vi "Error Query.vi"(8 "error in (no error)":errorcluster, 11 "VISA resource name":refnum<visa-resource-name>) -> (0 "error out":errorcluster, 1 "Error Message":string, 2 "Error Code":i32[](array[numeric]), 3 "VISA resource name out":refnum<visa-resource-name>)   [LabVIEW 2018, in "LeCroy Wave Series.lvlib"]
doc: "This VI queries the instrument for any errors in the instrument's error queue. It will continue to read errors until all errors have been read from the instrument. Any errors will be returned in the Error Out cluster.\n\nNote:\nThis VI is called automatically by most driver VIs so it is not usually necessary to call this in an application."
uses:
  LeCroy Wave Series.lvlib
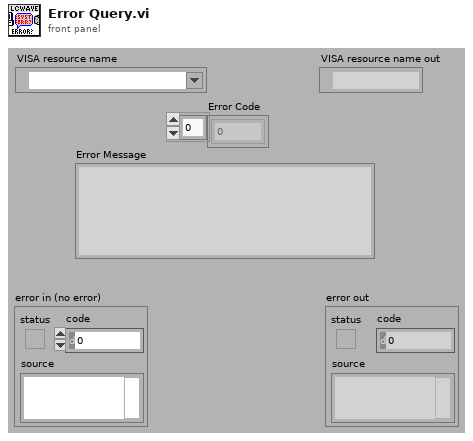
[diagram p1: front panel]
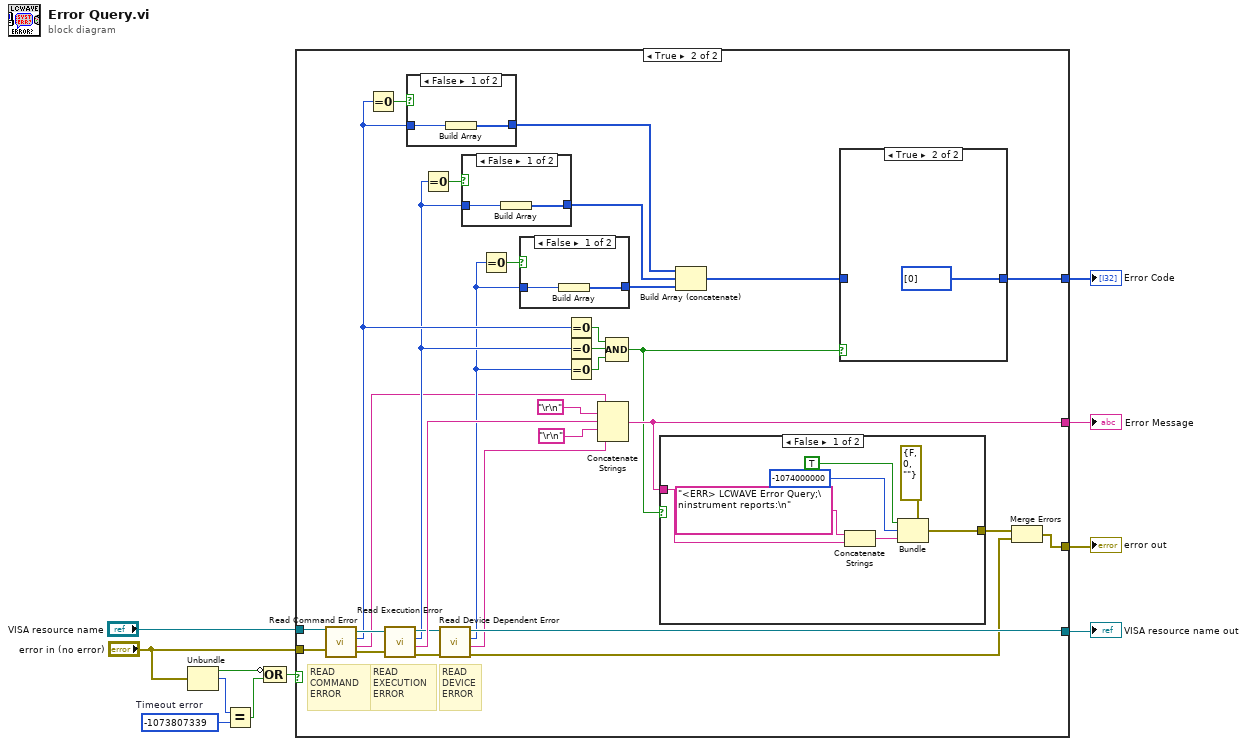
[diagram p0: block diagram]
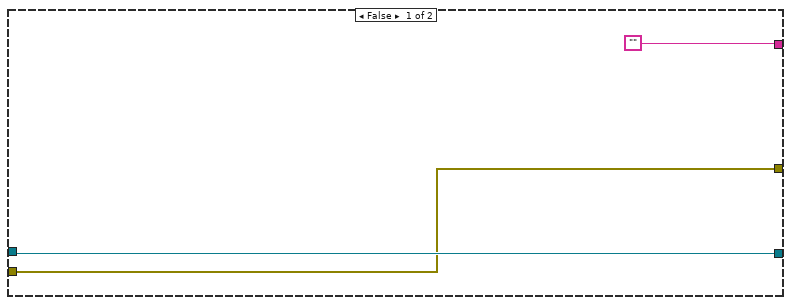
[diagram p2: hidden frame]
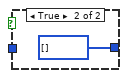
[diagram p4: hidden frame]
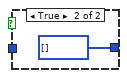
[diagram p5: hidden frame]
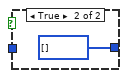
[diagram p6: hidden frame]
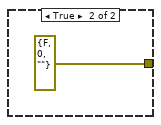
[diagram p7: hidden frame]
diagram:
  w4 = -1073807339  # Timeout error
  n1 = Unbundle("error in (no error)") -> ("status"=w6:bool, "code"=w5:i32)  [unwired: 1 out]
  n2 = Equal?(x=w5, y=w4) -> (x = y?=w3:bool)
  n3 = Compound Arithmetic op=OR(invert w6, w3) -> (w2:bool)
  n4 = case shown="True" w2 {
    tunnel: "VISA resource name" -> [w14 w39]
    tunnel: [w14 w32] -> w10
    tunnel: [w13 w40] -> w9
    tunnel: ["" ("Empty String Constant") w28] -> w8
    tunnel: "error in (no error)" -> [w13 w38]
    tunnel: [_ w17] -> w1
    frame False {
    }
    frame True {
      # "READ\nDEVICE\nERROR"
      # "READ\nEXECUTION\nERROR"
      # "READ\nCOMMAND\nERROR"
      n5 = call "Read Command Error.vi"("error in (no error)"=w38, "VISA resource name"=w39) -> ("error out"=w36:errorcluster, "Error Message"=w15:string, "Error Code"=w26:i32, "VISA resource name out"=w37:refnum<visa-resource-name>)  [unwired: 6 in]
      n6 = Equal To 0?(x=w26) -> (x = 0?=w27:bool)
      n7 = call "Read Execution Error.vi"("error in (no error)"=w36, "VISA resource name"=w37) -> ("error out"=w33:errorcluster, "Error Message"=w35:string, "Error Code"=w24:i32, "VISA resource name out"=w34:refnum<visa-resource-name>)  [unwired: 6 in]
      n8 = case shown="False" w27 {
        tunnel: [w54 i32[] []] -> w20
        tunnel: w26 -> [w55 _]
        frame False {
          n9 = Build Array(w55) -> (w54:i32[])
        }
        frame True {
        }
      }
      n10 = Equal To 0?(x=w24) -> (x = 0?=w25:bool)
      n11 = call "Read Device Dependent Error.vi"("error in (no error)"=w33, "VISA resource name"=w34) -> ("error out"=w31:errorcluster, "Error Message"=w29:string, "Error Code"=w22:i32, "VISA resource name out"=w32:refnum<visa-resource-name>)  [unwired: 6 in]
      n12 = case shown="False" w25 {
        tunnel: [w51 i32[] []] -> w19
        tunnel: w24 -> [w52 _]
        frame False {
          n13 = Build Array(w52) -> (w51:i32[])
        }
        frame True {
        }
      }
      n14 = Equal To 0?(x=w22) -> (x = 0?=w23:bool)
      n15 = case shown="False" w23 {
        tunnel: [w48 i32[] []] -> w18
        tunnel: w22 -> [w49 _]
        frame False {
          n16 = Build Array(w49) -> (w48:i32[])
        }
        frame True {
        }
      }
      n17 = Equal To 0?(x=w26) -> (x = 0?=w44:bool)
      n18 = Equal To 0?(x=w24) -> (x = 0?=w43:bool)
      n19 = Equal To 0?(x=w22) -> (x = 0?=w42:bool)
      n20 = Concatenate Strings(w15, "\r\n" ("End of Line Constant"), w35, "\r\n" ("End of Line Constant"), w29) -> (w28:string)
      n21 = Compound Arithmetic op=AND(w44, w43, w42) -> (w21:bool)
      n22 = case shown="False" w21 {
        tunnel: w28 -> [w62 _]
        tunnel: [w57 errorcluster {"status"=FALSE, "code"=0, "source"=""} ("error out")] -> w41
        frame False {
          n23 = Concatenate Strings("<ERR> LCWAVE Error Query;\ninstrument reports:\n" ("Source"), w62) -> (w59:string)
          n24 = Bundle(cluster=errorcluster {"status"=FALSE, "code"=0, "source"=""} ("error out"), "status"=TRUE, "code"=-1074000000 ("Code"), "source"=w59) -> (w57:errorcluster)
        }
        frame True {
        }
      }
      n25 = Build Array (concatenate)(w20, w19, w18) -> (w16:i32[])
      n26 = case shown="True" w21 {
        tunnel: [w46 i32[] [0]] -> w17
        tunnel: w16 -> [w46 _]
        frame False {
        }
        frame True {
        }
      }
      n27 = Merge Errors(w41, w31) -> (w40:errorcluster)
    }
  }
  "VISA resource name out" <- w10
  "error out" <- w9
  "Error Message" <- w8
  "Error Code" <- w1
